vi "chart.vi"() -> ()   [LabVIEW 2010]
uses:
  <vilib>/Instr/_visa.llb/VISA Configure Serial Port (Instr).vi
panel:
  out "Orientation Z":dbl(knob) scale=-90.0..90.0
  out "Orientation Y":dbl(knob) scale=-90.0..90.0
  out "Orientation X":dbl(knob) scale=0.0..360.0
  out "output cluster 2":cluster{dbl, dbl, dbl}
  out "Orientation":cluster{dbl, dbl, dbl}(graph)
  out "output cluster":cluster{dbl, dbl, dbl}
  out "Acceleration":cluster{dbl, dbl, dbl}(graph)
  out "SYNC received":bool
  out "line":string
  in  "stop":bool
  out "read buffer":string
  out "Serial Settings:Number of Bytes at Serial Port":u32
  in  "VISA resource name":refnum<visa-resource-name>
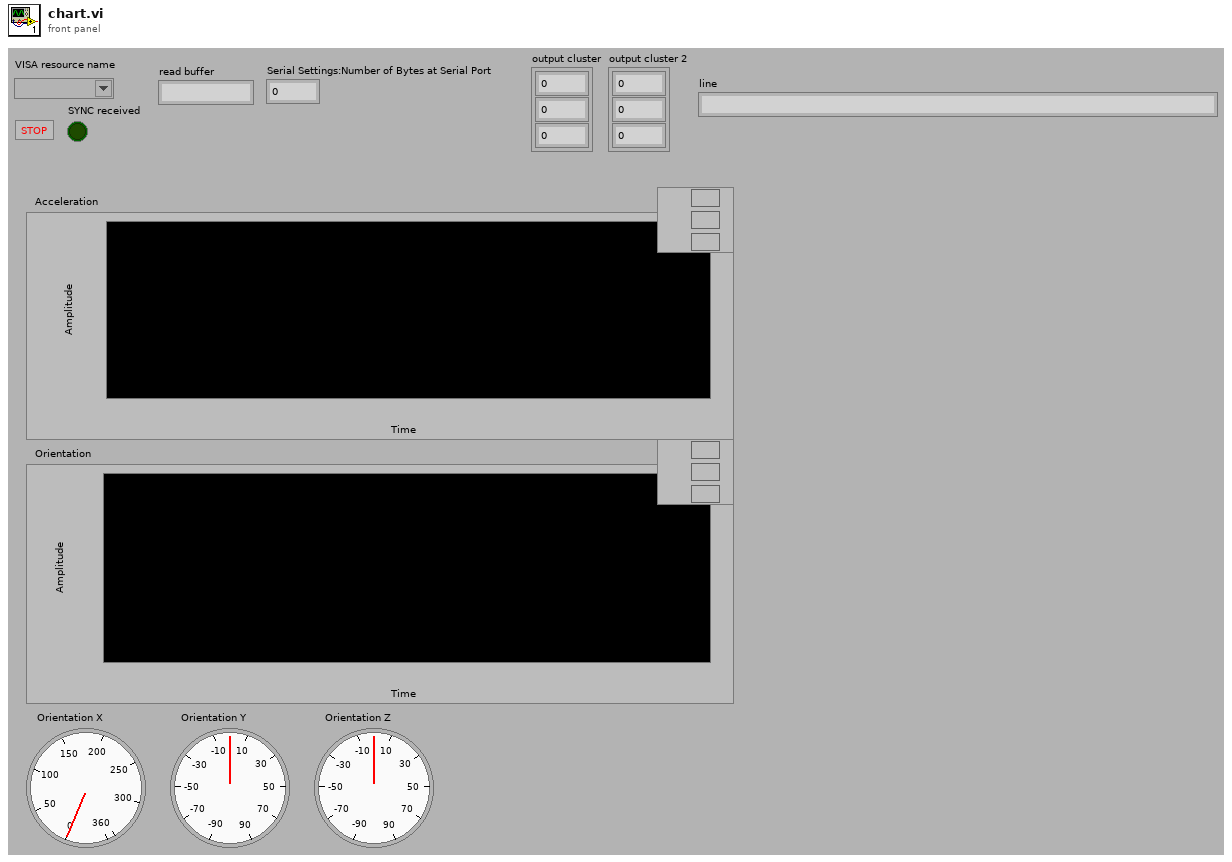
[diagram p1: front panel]
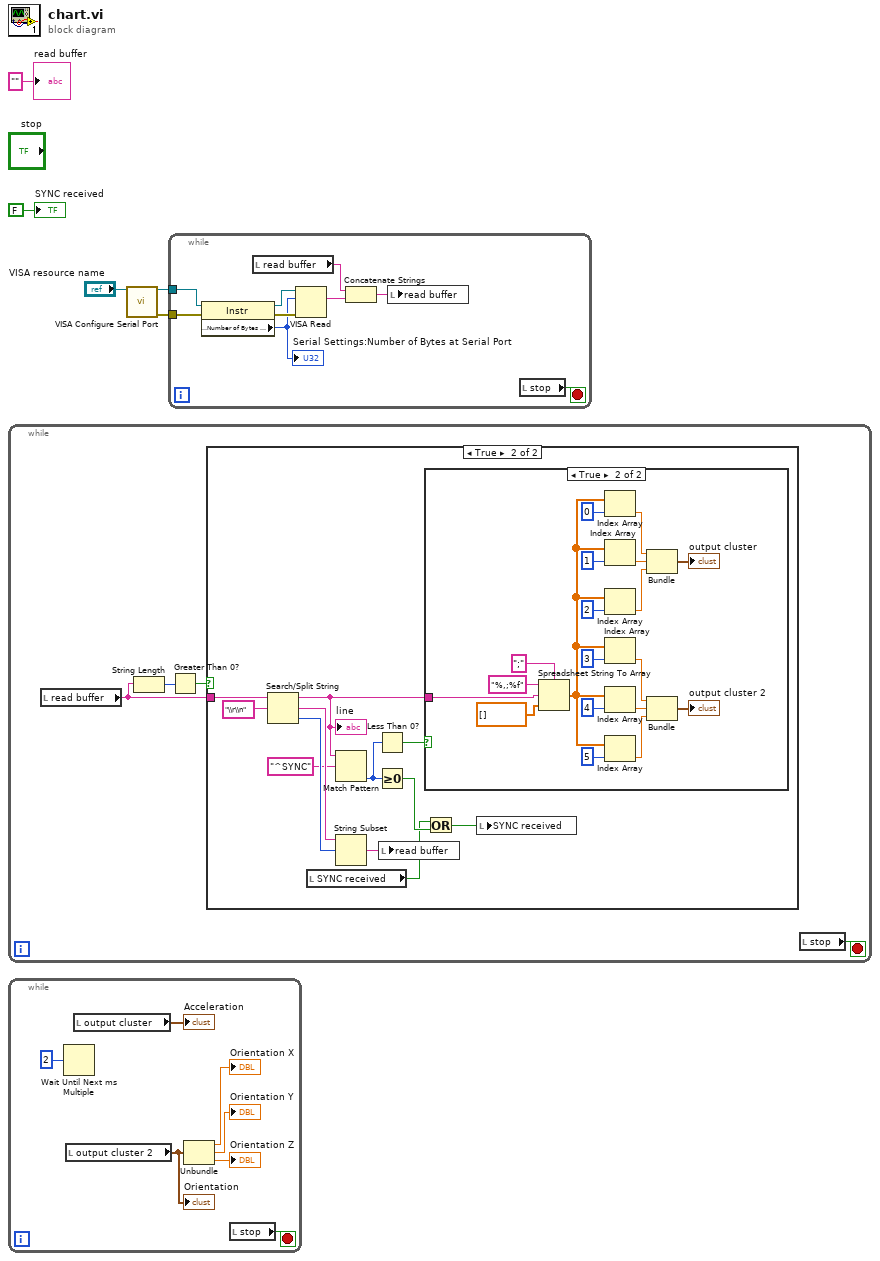
[diagram p0: block diagram]
diagram:
  n1 = while {
    stop <- w9 stop-if-true
    n2 = local read "read buffer"() -> (w6:string)
    n3 = String Length(string=w6) -> (length=w8:i32)
    n4 = Greater Than 0?(x=w8) -> (x > 0?=w7:bool)
    n5 = case shown="True" w7 {
      tunnel: w6 -> [_ w21]
      frame False {
      }
      frame True {
        n6 = Search/Split String(string=w21, search string/char (-)="\\r\\n") -> (substring before match=w10:string, match + rest of string=w19:string, offset of match=w18:i32)  [unwired: 1 in]
        "line" <- w10
        n7 = local read "SYNC received"() -> (w14:bool)
        n8 = Match Pattern(string=w10, regular expression="^SYNC") -> (offset past match=w11:i32)  [unwired: 1 in, 3 out]
        n9 = String Subset(string=w19, offset (0)=w18) -> (substring=w17:string)  [unwired: 1 in]
        n10 = Less Than 0?(x=w11) -> (x < 0?=w12:bool)
        n11 = Greater Or Equal To 0?(x=w11) -> (x >= 0?=w15:bool)
        n12 = local write "read buffer"(w17) -> ()
        n13 = case shown="True" w12 {
          tunnel: w10 -> [_ w38]
          frame False {
          }
          frame True {
            n14 = Spreadsheet String To Array(delimiter (Tab)=";", format string="%,;%f", spreadsheet string=w38, array type (2D Dbl)=dbl[] []) -> (array=w26:dbl[])
            n15 = Index Array(array=w26, index=0 ("index (row)")) -> (element=w33:dbl)
            n16 = Index Array(array=w26, index=1 ("index (row)")) -> (element=w31:dbl)
            n17 = Index Array(array=w26, index=2 ("index (row)")) -> (element=w32:dbl)
            n18 = Index Array(array=w26, index=3 ("index (row)")) -> (element=w25:dbl)
            n19 = Index Array(array=w26, index=4 ("index (row)")) -> (element=w24:dbl)
            n20 = Index Array(array=w26, index=5 ("index (row)")) -> (element=w23:dbl)
            n21 = Bundle(w33, w31, w32) -> (→"output cluster":cluster{dbl, dbl, dbl})  [unwired: 1 in]
            n22 = Bundle(w25, w24, w23) -> (→"output cluster 2":cluster{dbl, dbl, dbl})  [unwired: 1 in]
          }
        }
        n23 = Or(x=w14, y=w15) -> (x .or. y?=w13:bool)
        n24 = local write "SYNC received"(w13) -> ()
      }
    }
    n25 = local read "stop"() -> (w9:bool)
  }
  n26 = while {
    stop <- w47 stop-if-true
    n27 = Wait Until Next ms Multiple(millisecond multiple=u32 2) -> ()  [unwired: 1 out]
    n28 = local read "output cluster 2"() -> (w44:cluster{dbl, dbl, dbl})
    "Orientation" <- w44
    n29 = local read "output cluster"() -> (→"Acceleration":cluster{dbl, dbl, dbl})
    n30 = Unbundle(w44) -> (→"Orientation X":dbl, →"Orientation Y":dbl, →"Orientation Z":dbl)
    n31 = local read "stop"() -> (w47:bool)
  }
  n32 = call-poly "VISA Configure Serial Port"("VISA resource name"="VISA resource name") -> ("VISA resource name out"=w4:refnum<visa-resource-name>, "error out"=w3:errorcluster)  [unwired: 13 in]
  n33 = while {
    tunnel: w4 -> [w55]
    tunnel: w3 -> [w56]
    stop <- w48 stop-if-true
    n34 = property class="Instr"(reference=w55, error in=w56) -> (reference out=w54:refnum<visa-resource-name>, error out=w53:errorcluster, "Serial Settings:Number of Bytes at Serial Port"=w52:u32)
    "Serial Settings:Number of Bytes at Serial Port" <- w52
    n35 = local read "read buffer"() -> (w50:string)
    n36 = VISA Read(VISA resource name=w54, byte count=w52, error in (no error)=w53) -> (read buffer=w49:string)  [unwired: 3 out]
    n37 = Concatenate Strings(w50, w49) -> (w51:string)
    n38 = local write "read buffer"(w51) -> ()
    n39 = local read "stop"() -> (w48:bool)
  }
  "read buffer" <- "" ("read buffer")
  "SYNC received" <- FALSE ("SYNC received")
